vi "main 0.3.vi"() -> ()   [LabVIEW 2012]
uses:
  <vilib>/Utility/file.llb/Write To Spreadsheet File (DBL).vi
  <vilib>/Analysis/1siggen.llb/Ramp Pattern by Samples.vi
  <vilib>/Analysis/NI_AALBase.lvlib
panel:
  in  "stop":bool
  out "Slide":dbl(slide) scale=0.0..1.0
  in  "Tab Control":enum32{"live", "XY"}(tab)
  in  "binning":dbl=4.0
  in  "exp time [s]":dbl=0.01
  in  "frames":i32=1
  in  "avg[t] acc[f]":bool
  in  "threshold":i32=1
  in  "dark?":bool
  in  "dark":bool
  out "Waveform Chart":dbl(graph)=418707489.0
  in  "snap":bool
  in  "count?":bool
  in  "save":bool
  in  "Path":path
  out "XY":dbl[][](graph)
  in  "meas_start_XY":bool
  in  "Axis2":string(combo)="4D Z"
  in  "Axis1":string(combo)="4D Z"
  in  "windows":dbl=1000.0 caption="+/- window" format="%#_6e"
  in  "steps":u32=10
  in  "IP address":string="172.24.192.135"
  in  "meas_stop_XY":bool
  out "captured":dbl[][](graph)
  out "live":dbl[][](graph)
  in  "close":bool
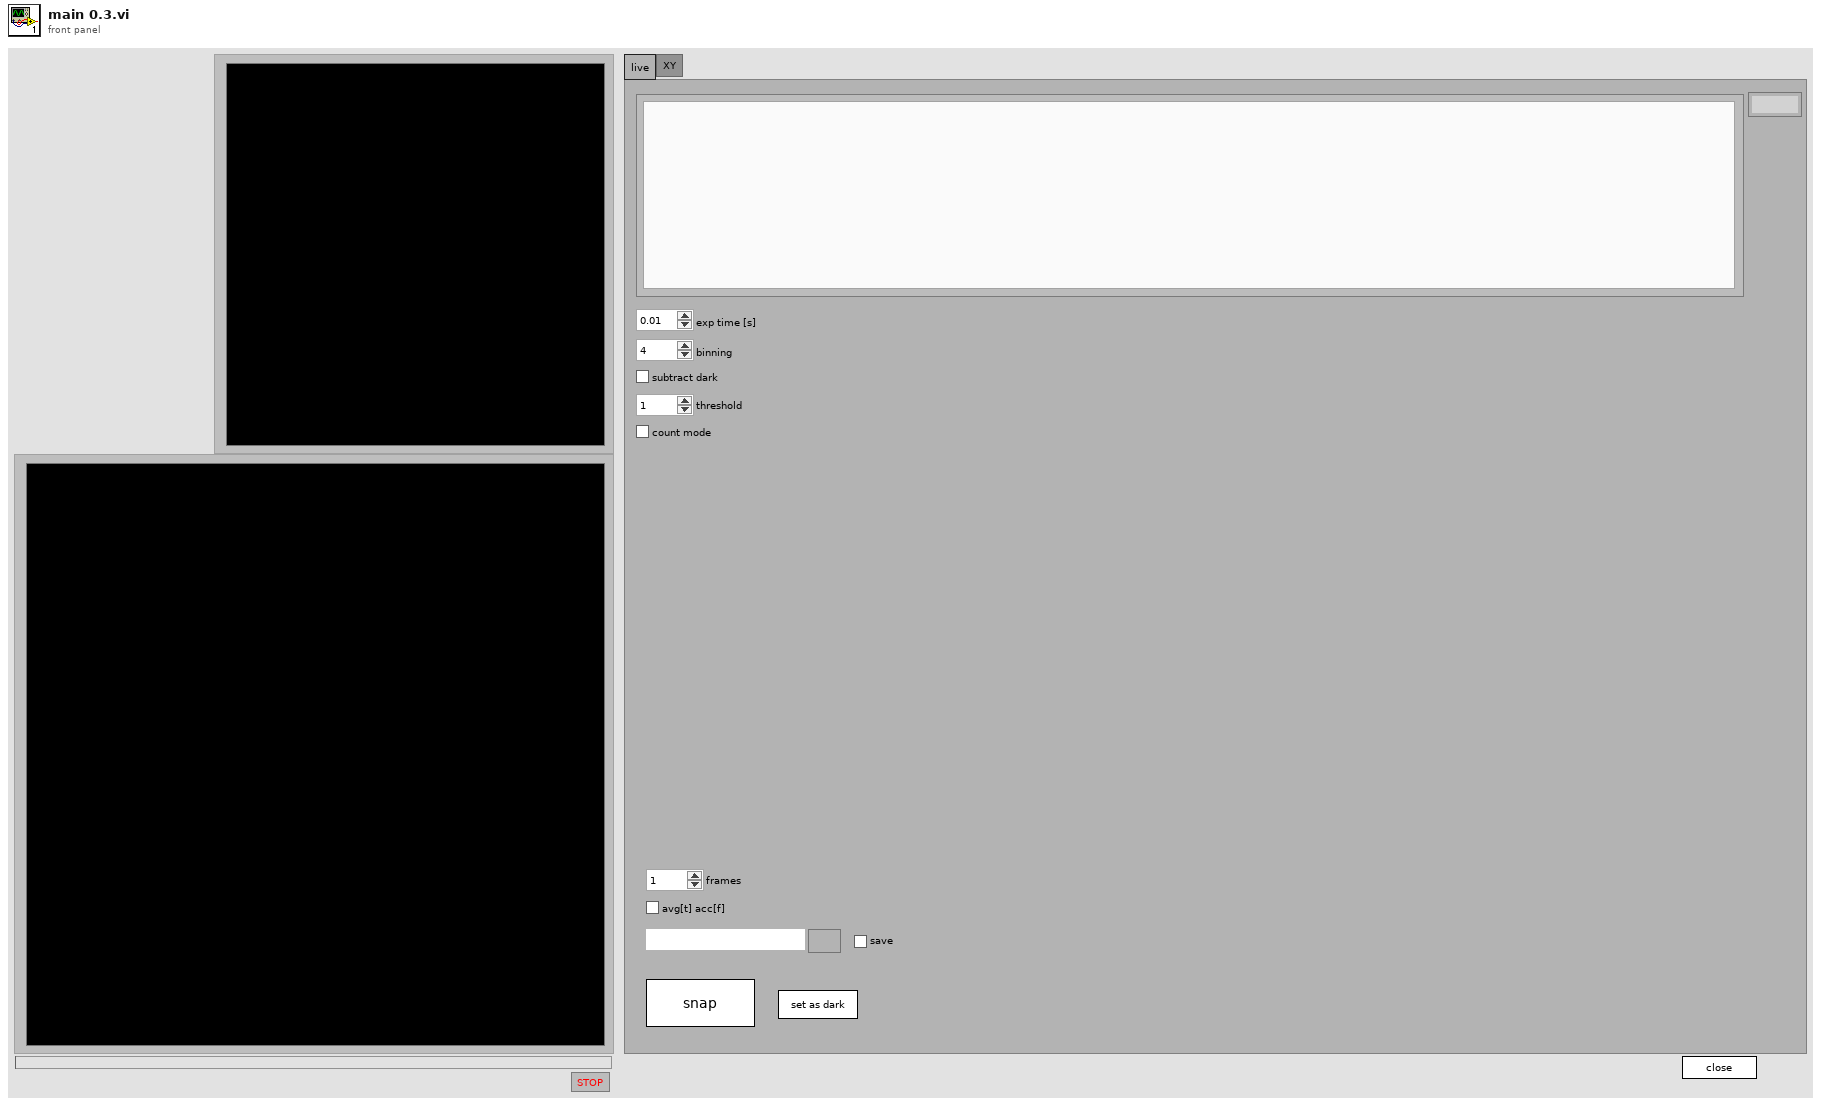
[diagram p1: front panel]
types:
  T1 = cluster{"height":u32, "width":u32, "datatype":u32}
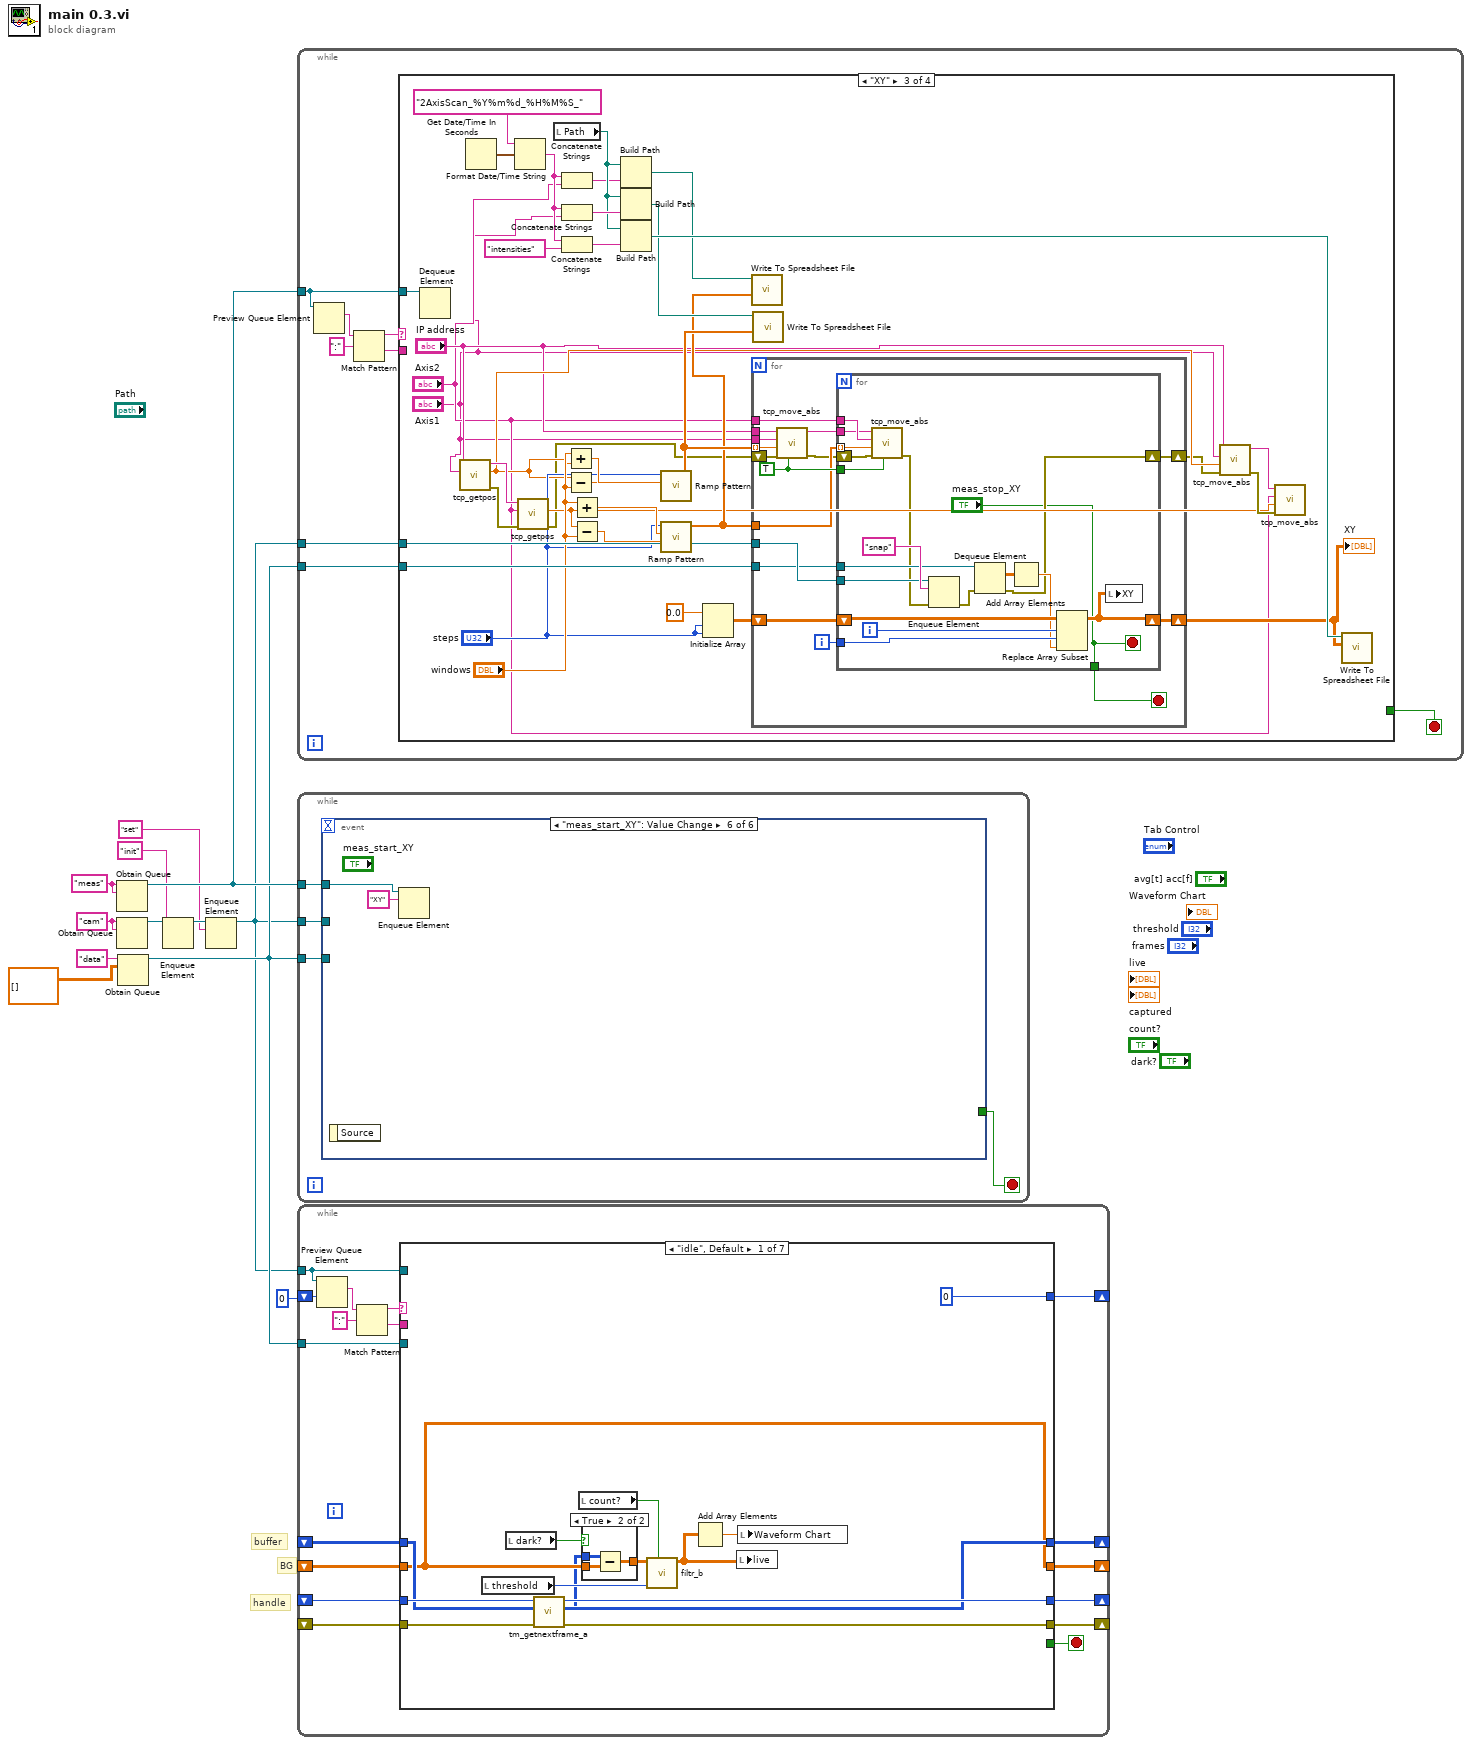
[diagram p0: block diagram]
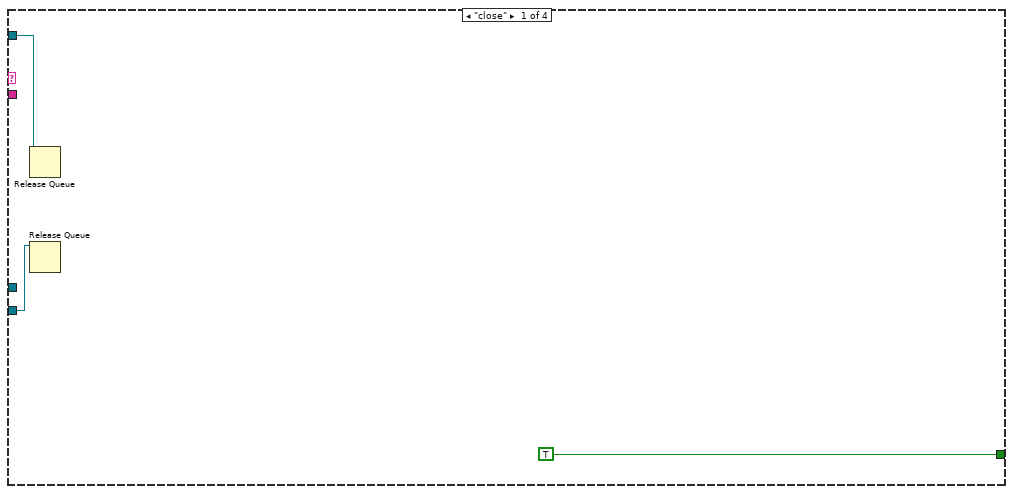
[diagram p2: hidden frame]
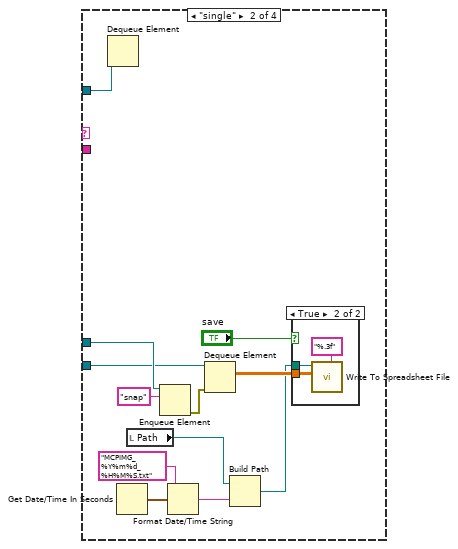
[diagram p3: hidden frame]
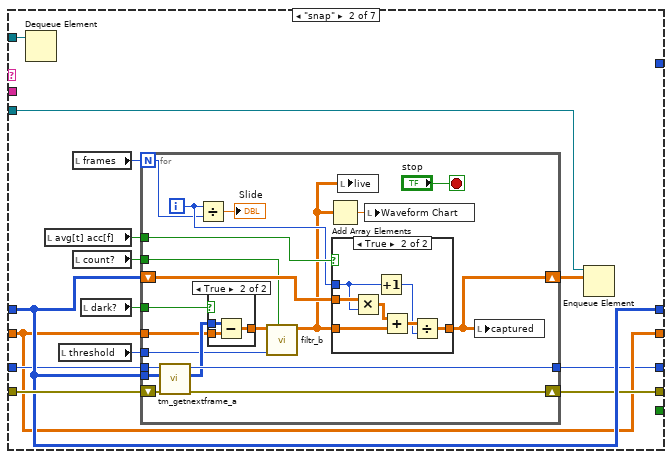
[diagram p7: hidden frame]
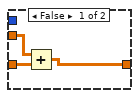
[diagram p8: hidden frame]
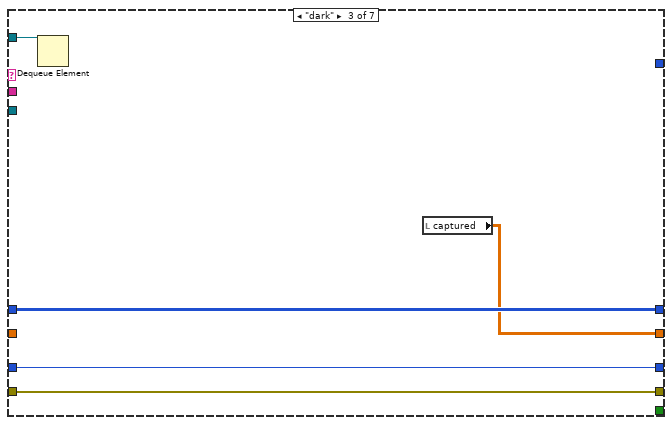
[diagram p10: hidden frame]
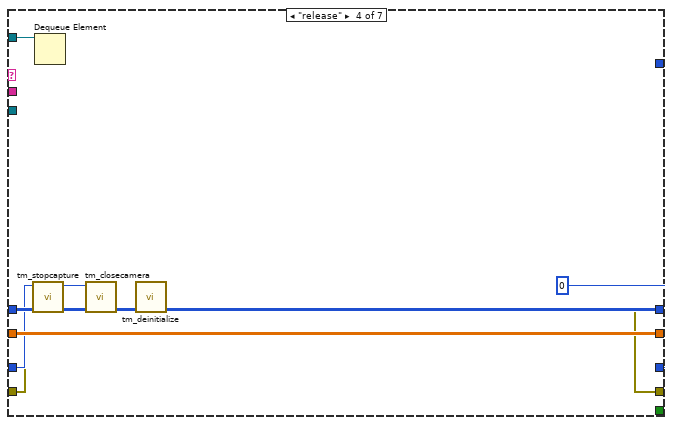
[diagram p11: hidden frame]
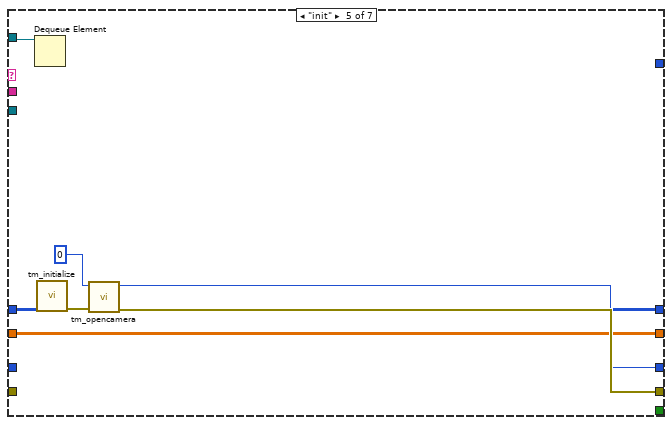
[diagram p12: hidden frame]
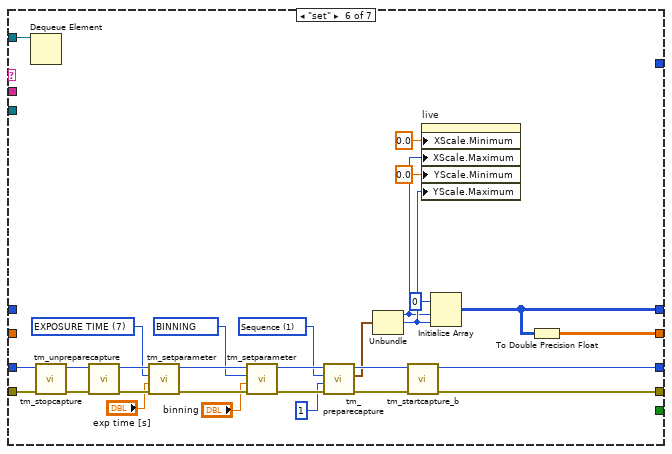
[diagram p13: hidden frame]
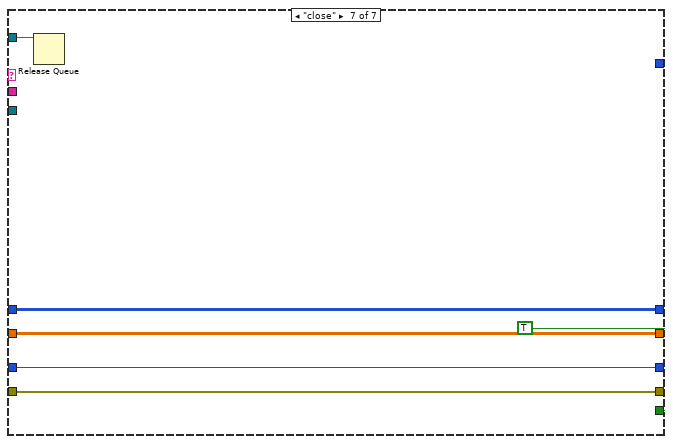
[diagram p14: hidden frame]
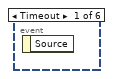
[diagram p15: hidden frame]
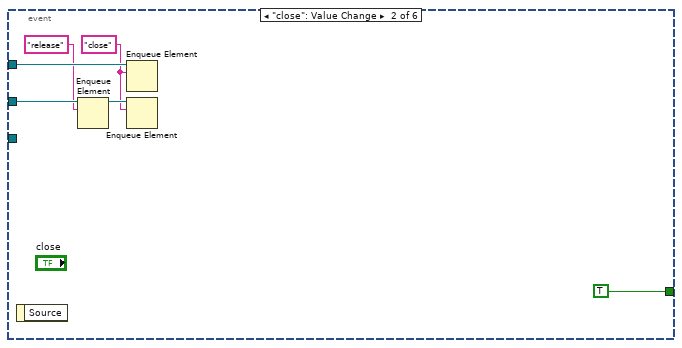
[diagram p16: hidden frame]
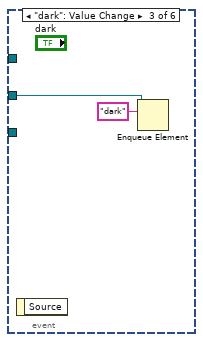
[diagram p17: hidden frame]
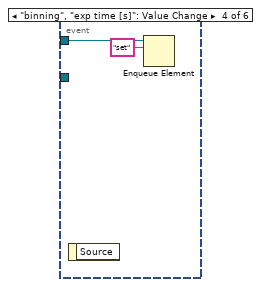
[diagram p18: hidden frame]
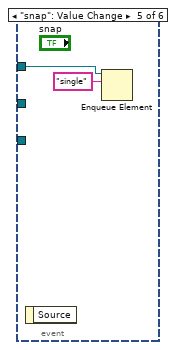
[diagram p19: hidden frame]
diagram:
  w9 = "meas" ("name (unnamed)")
  w10 = "cam" ("name (unnamed)")
  # "BG"
  # "handle"
  # "buffer"
  n1 = Obtain Queue(name (unnamed)=w9, element data type=w9) -> (queue out=w8:refnum<queue>)  [unwired: 3 in, 2 out]
  n2 = Obtain Queue(name (unnamed)=w10, element data type=w10) -> (queue out=w12:refnum<queue>)  [unwired: 3 in, 2 out]
  n3 = Obtain Queue(name (unnamed)="data", element data type=dbl[][] []) -> (queue out=w2:refnum<queue>)  [unwired: 3 in, 2 out]
  n4 = Enqueue Element(queue=w12, element="init") -> (queue out=w6:refnum<queue>)  [unwired: 2 in, 2 out]
  n5 = Enqueue Element(queue=w6, element="set") -> (queue out=w1:refnum<queue>)  [unwired: 2 in, 2 out]
  n6 = while {
    tunnel: w8 -> [w16]
    tunnel: w2 -> [w15]
    tunnel: w1 -> [w13]
    stop <- w14 stop-if-true
    n7 = Preview Queue Element(queue=w16) -> (element=w20:string)  [unwired: 2 in, 3 out]
    n8 = Match Pattern(string=w20, regular expression=":") -> (before substring=w18:string, after substring=w17:string)  [unwired: 1 in, 2 out]
    n9 = case shown="\"XY\"" w18 {
      tunnel: w17 -> [_ _ _ _]
      tunnel: w16 -> [w22 w35 w74 _]
      tunnel: w15 -> [w23 w32 w70 _]
      tunnel: [TRUE _ _ _] -> w14
      tunnel: w13 -> [_ w34 w71 _]
      frame "close" {
        n10 = Release Queue(queue=w22) -> ()  [unwired: 2 in, 3 out]
        n11 = Release Queue(queue=w23) -> ()  [unwired: 2 in, 3 out]
      }
      frame "single" {
        n12 = Dequeue Element(queue=w35) -> ()  [unwired: 2 in, 4 out]
        n13 = Get Date/Time In Seconds() -> (seconds since 1Jan1904=w28:timestamp)
        n14 = local read "Path"() -> (w24:path)
        n15 = Enqueue Element(queue=w34, element="snap") -> (error out=w31:errorcluster)  [unwired: 2 in, 2 out]
        n16 = Format Date/Time String(time format string (%c)="MCPIMG_%Y%m%d_%H%M%S.txt", seconds (now)=w28) -> (date/time string=w26:string)  [unwired: 1 in]
        n17 = Dequeue Element(queue=w32, error in (no error)=w31) -> (element=w30:dbl[][])  [unwired: 1 in, 3 out]
        n18 = Build Path(base path=w24, name or relative path=w26) -> (appended path=w25:path)
        n19 = case shown="True" "save" {
          tunnel: w30 -> [_ w38]
          tunnel: w25 -> [_ w36]
          frame False {
          }
          frame True {
            n20 = call-poly <vilib>:"Write To Spreadsheet File.vi"("format (%.3f)"="%.3f", "2D data"=w38, "file path (dialog if empty)"=w36) -> ()  [unwired: 5 in, 1 out]
          }
        }
      }
      frame "XY" {
        n21 = Dequeue Element(queue=w74) -> ()  [unwired: 2 in, 4 out]
        n22 = call "tcp_getpos.vi"("Axis"="Axis1", "IP address"="IP address") -> ("error out"=w58:errorcluster, "position"=w45:dbl, "IP address out"=w59:string)  [unwired: 7 in]
        n23 = Get Date/Time In Seconds() -> (seconds since 1Jan1904=w69:timestamp)
        n24 = Format Date/Time String(time format string (%c)="2AxisScan_%Y%m%d_%H%M%S_", seconds (now)=w69) -> (date/time string=w53:string)  [unwired: 1 in]
        n25 = call "tcp_getpos.vi"("error in (no error)"=w58, "Axis"="Axis2", "IP address"=w59) -> ("error out"=w39:errorcluster, "position"=w43:dbl)  [unwired: 6 in, 1 out]
        n26 = local read "Path"() -> (w52:path)
        n27 = Concatenate Strings(w53, "Axis2") -> (w51:string)
        n28 = Concatenate Strings(w53, "Axis1") -> (w65:string)
        n29 = Concatenate Strings(w53, "intensities" ("name or relative path")) -> (w66:string)
        n30 = Add(x="windows", y=w45) -> (x+y=w61:dbl)
        n31 = Subtract(x=w45, y="windows") -> (x-y=w60:dbl)
        n32 = Add(x="windows", y=w43) -> (x+y=w56:dbl)
        n33 = Subtract(x=w43, y="windows") -> (x-y=w55:dbl)
        n34 = Build Path(base path=w52, name or relative path=w51) -> (appended path=w50:path)
        n35 = Build Path(base path=w52, name or relative path=w65) -> (appended path=w62:path)
        n36 = Build Path(base path=w52, name or relative path=w66) -> (appended path=w64:path)
        n37 = call-poly <vilib>:"Ramp Pattern.vi"("start"=w60, "end"=w61, "samples"="steps") -> ("Ramp Pattern"=w63:dbl[])  [unwired: 7 in, 1 out]
        n38 = call-poly <vilib>:"Ramp Pattern.vi"("start"=w55, "end"=w56, "samples"="steps") -> ("Ramp Pattern"=w49:dbl[])  [unwired: 7 in, 1 out]
        n39 = Initialize Array(0.0 ("element"), "steps", "steps") -> (w72:dbl[][])
        n40 = call-poly <vilib>:"Write To Spreadsheet File.vi"("1D data"=w49, "file path (dialog if empty)"=w50) -> ()  [unwired: 6 in, 1 out]
        n41 = for {
          tunnel: w63 -> [w90] mode=indexing
          tunnel: "Axis1" -> [w89]
          tunnel: w71 -> [w88]
          tunnel: w70 -> [w87]
          tunnel: "Axis2" -> [w83]
          tunnel: "IP address" -> [w82]
          shift-right: [w81] -> w48
          shift-left: w72 -> [w86]
          tunnel: w49 -> [w80]
          shift-right: [w77] -> w40
          shift-left: w39 -> [w76]
          i -> [w85]
          stop <- w75 stop-if-true
          w84 = TRUE ("wait4motiondone")
          n42 = call "tcp_move_abs.vi"("wait4motiondone"=w84, "error in (no error)"=w76, "destination nm/u°"=w90, "Axis"=w89, "IP address"=w82) -> ("error out"=w79:errorcluster, "IP address out"=w78:string)  [unwired: 4 in, 1 out]
          n43 = for {
            tunnel: w80 -> [w99] mode=indexing
            tunnel: w88 -> [w106]
            tunnel: w87 -> [w105]
            tunnel: w85 -> [w103]
            shift-right: [w93] -> w81
            shift-left: w86 -> [w104]
            tunnel: w84 -> [w97]
            tunnel: w83 -> [w96]
            tunnel: w78 -> [w94]
            shift-right: [w92] -> w77
            shift-left: w79 -> [w95]
            tunnel: ["meas_stop_XY"] -> w75
            i -> [w102]
            stop <- "meas_stop_XY" stop-if-true
            n44 = call "tcp_move_abs.vi"("wait4motiondone"=w97, "error in (no error)"=w95, "destination nm/u°"=w99, "Axis"=w96, "IP address"=w94) -> ("error out"=w98:errorcluster)  [unwired: 4 in, 2 out]
            n45 = Enqueue Element(queue=w106, element="snap", error in (no error)=w98) -> (error out=w107:errorcluster)  [unwired: 1 in, 2 out]
            n46 = Dequeue Element(queue=w105, error in (no error)=w107) -> (element=w101:dbl[][], error out=w92:errorcluster)  [unwired: 1 in, 2 out]
            n47 = Add Array Elements(numeric array=w101) -> (sum=w100:dbl)
            n48 = Replace Array Subset(array=w104, new element=w100, index (row)=w102, index (col)=w103) -> (w93:dbl[][])
            n49 = local write "XY"(w93) -> ()
          }
        }
        "XY" <- w48
        n50 = call-poly <vilib>:"Write To Spreadsheet File.vi"("1D data"=w63, "file path (dialog if empty)"=w62) -> ()  [unwired: 6 in, 1 out]
        n51 = call "tcp_move_abs.vi"("error in (no error)"=w40, "destination nm/u°"=w45, "Axis"="Axis1", "IP address"="IP address") -> ("error out"=w47:errorcluster, "IP address out"=w46:string)  [unwired: 5 in, 1 out]
        n52 = call "tcp_move_abs.vi"("error in (no error)"=w47, "destination nm/u°"=w43, "Axis"="Axis2", "IP address"=w46) -> ()  [unwired: 5 in, 3 out]
        n53 = call-poly <vilib>:"Write To Spreadsheet File.vi"("2D data"=w48, "file path (dialog if empty)"=w64) -> ()  [unwired: 6 in, 1 out]
      }
      frame "idle", Default {
      }
    }
  }
  n54 = while {
    tunnel: w1 -> [w112]
    tunnel: w8 -> [w111]
    tunnel: w2 -> [w110]
    stop <- w109 stop-if-true
    n55 = event shown="[5] \"meas_start_XY\": Value Change" {
      selector: _ -> [_ _ _ _ _ _]
      dyn-events: _ -> [_ _ _ _ _ _]
      timeout: _ -> [_ _ _ _ _ _]
      tunnel: w112 -> [_ w117 w120 w122 _ _]
      tunnel: w111 -> [_ w118 _ _ w123 w125]
      tunnel: w110 -> [_ _ _ _ _ _]
      tunnel: [_ TRUE _ _ _ _] -> w109
      event Timeout {
        n56 = event-data() -> ()  [unwired: 1 in, 1 out]
      }
      event "close": Value Change {
        w114 = "close" ("element")
        n57 = event-data() -> ()  [unwired: 1 in, 1 out]
        n58 = Enqueue Element(queue=w117, element="release") -> (queue out=w116:refnum<queue>)  [unwired: 2 in, 2 out]
        n59 = Enqueue Element(queue=w118, element=w114) -> ()  [unwired: 2 in, 3 out]
        n60 = Enqueue Element(queue=w116, element=w114) -> ()  [unwired: 2 in, 3 out]
      }
      event "dark": Value Change {
        n61 = event-data() -> ()  [unwired: 1 in, 1 out]
        n62 = Enqueue Element(queue=w120, element="dark") -> ()  [unwired: 2 in, 3 out]
      }
      event "binning", "exp time [s]": Value Change {
        n63 = event-data() -> ()  [unwired: 1 in, 1 out]
        n64 = Enqueue Element(queue=w122, element="set") -> ()  [unwired: 2 in, 3 out]
      }
      event "snap": Value Change {
        n65 = event-data() -> ()  [unwired: 1 in, 1 out]
        n66 = Enqueue Element(queue=w123, element="single") -> ()  [unwired: 2 in, 3 out]
      }
      event "meas_start_XY": Value Change {
        n67 = event-data() -> ()  [unwired: 1 in, 1 out]
        n68 = Enqueue Element(queue=w125, element="XY") -> ()  [unwired: 2 in, 3 out]
      }
    }
  }
  n69 = while {
    tunnel: w1 -> [w139]
    shift-right: [w137] -> _
    shift-left: _ -> [w136]
    shift-right: [w135] -> _
    shift-left: _ -> [w134]
    shift-right: [w133] -> _
    shift-left: _ -> [w132]
    shift-right: [w131] -> _
    shift-left: _ -> [w130]
    shift-right: [w128] -> _
    shift-left: 0 -> [w129]
    tunnel: w2 -> [w127]
    stop <- w138 stop-if-true
    n70 = Preview Queue Element(queue=w139, timeout in ms (-1)=w129) -> (element=w143:string)  [unwired: 1 in, 3 out]
    n71 = Match Pattern(string=w143, regular expression=":") -> (before substring=w141:string, after substring=w140:string)  [unwired: 1 in, 2 out]
    n72 = case shown="\"idle\", Default" w141 {
      tunnel: w140 -> [_ _ _ _ _ _ _]
      tunnel: w139 -> [_ w167 w214 w224 w225 w237 w266]
      tunnel: [_ _ _ _ _ _ TRUE] -> w138
      tunnel: [w152 w169 w212 w216 w230 w238 w261] -> w137
      tunnel: w136 -> [w154 w172 w212 w220 _ w260 w261]
      tunnel: [w153 w164 w211 u32 0 ("Handle out") w228 w239 w262] -> w135
      tunnel: w134 -> [w155 w170 w211 w221 _ w258 w262]
      tunnel: [w151 w171 w213 w222 w226 w240 w263] -> w133
      tunnel: w132 -> [w151 w171 w213 w222 w226 _ w263]
      tunnel: [w150 w168 w210 w223 w227 w241 w264] -> w131
      tunnel: w130 -> [w150 w168 _ w223 w227 _ w264]
      tunnel: [0 _ _ _ _ _ _] -> w128
      tunnel: w127 -> [_ w163 _ _ _ _ _]
      frame "idle", Default {
        n73 = local read "threshold"() -> (w156:i32)
        n74 = local read "dark?"() -> (w157:bool)
        n75 = call "tm_getnextframe_a.vi"("error in (no error)"=w154, "Buffer"=w151, "Handle in"=w155) -> ("error out"=w152:errorcluster, "Data"=w148:u16[][], "Handle out"=w153:u32)  [unwired: 6 in]
        n76 = local read "count?"() -> (w146:bool)
        n77 = case shown="True" w157 {
          tunnel: [w158 w161] -> w147
          tunnel: w148 -> [w158 w160]
          tunnel: w150 -> [_ w159]
          frame False {
          }
          frame True {
            n78 = Subtract(x=w160, y=w159) -> (x-y=w161:dbl[][])
          }
        }
        n79 = call "filtr_b.vi"("count?"=w146, "threshold"=w156, "input array"=w147) -> ("output array"=w145:dbl[][])  [unwired: 8 in]
        n80 = Add Array Elements(numeric array=w145) -> (sum=w144:dbl)
        n81 = local write "live"(w145) -> ()
        n82 = local write "Waveform Chart"(w144) -> ()
      }
      frame "snap" {
        n83 = Dequeue Element(queue=w167) -> ()  [unwired: 2 in, 4 out]
        n84 = local read "avg[t] acc[f]"() -> (w166:bool)
        n85 = local read "threshold"() -> (w174:i32)
        n86 = local read "frames"() -> (w173:i32)
        n87 = local read "count?"() -> (w165:bool)
        n88 = local read "dark?"() -> (w175:bool)
        n89 = for {
          N: w173 -> [w180]
          tunnel: w175 -> [w195]
          tunnel: w171 -> [w193]
          tunnel: w170 -> [w194]
          tunnel: w174 -> [w187]
          tunnel: [w191] -> w164
          shift-right: [w190] -> w169
          shift-left: w172 -> [w192]
          tunnel: w168 -> [w186]
          shift-right: [w183] -> w162
          shift-left: w171 -> [w184]
          tunnel: w166 -> [w185]
          tunnel: w165 -> [w182]
          i -> [w181]
          stop <- "stop" stop-if-true
          n90 = call "tm_getnextframe_a.vi"("error in (no error)"=w192, "Buffer"=w193, "Handle in"=w194) -> ("error out"=w190:errorcluster, "Data"=w189:u16[][], "Handle out"=w191:u32)  [unwired: 6 in]
          n91 = Divide(x=w181, y=w180) -> (x/y=→"Slide":dbl)
          n92 = case shown="True" w195 {
            tunnel: [w206 w209] -> w188
            tunnel: w189 -> [w206 w208]
            tunnel: w186 -> [_ w207]
            frame False {
            }
            frame True {
              n93 = Subtract(x=w208, y=w207) -> (x-y=w209:dbl[][])
            }
          }
          n94 = call "filtr_b.vi"("count?"=w182, "threshold"=w187, "input array"=w188) -> ("output array"=w177:dbl[][])  [unwired: 8 in]
          n95 = Add Array Elements(numeric array=w177) -> (sum=w178:dbl)
          n96 = case shown="True" w185 {
            tunnel: w184 -> [w198 w205]
            tunnel: w177 -> [w197 w203]
            tunnel: [w196 w199] -> w183
            tunnel: w181 -> [_ w200]
            frame False {
              n97 = Add(x=w198, y=w197) -> (x+y=w196:dbl[][])
            }
            frame True {
              n98 = Multiply(x=w205, y=w200) -> (x*y=w204:dbl[][])
              n99 = Increment(x=w200) -> (x+1=w201:i32)
              n100 = Add(x=w204, y=w203) -> (x+y=w202:dbl[][])
              n101 = Divide(x=w202, y=w201) -> (x/y=w199:dbl[][])
            }
          }
          n102 = local write "live"(w177) -> ()
          n103 = local write "Waveform Chart"(w178) -> ()
          n104 = local write "captured"(w183) -> ()
        }
        n105 = Enqueue Element(queue=w163, element=w162) -> ()  [unwired: 2 in, 3 out]
      }
      frame "dark" {
        n106 = Dequeue Element(queue=w214) -> ()  [unwired: 2 in, 4 out]
        n107 = local read "captured"() -> (w210:dbl[][])
      }
      frame "release" {
        n108 = call "tm_stopcapture.vi"("error in (no error)"=w220, "Handle in"=w221) -> ("error out"=w218:errorcluster, "Handle out"=w219:u32)  [unwired: 8 in]
        n109 = Dequeue Element(queue=w224) -> ()  [unwired: 2 in, 4 out]
        n110 = call "tm_closecamera.vi"("error in (no error)"=w218, "Handle in"=w219) -> ("error out"=w217:errorcluster)  [unwired: 9 in]
        n111 = call "tm_deinitialize.vi"("error in (no error)"=w217) -> ("error out"=w216:errorcluster)  [unwired: 10 in]
      }
      frame "init" {
        n112 = Dequeue Element(queue=w225) -> ()  [unwired: 2 in, 4 out]
        n113 = call "tm_initialize.vi"() -> ("error out"=w231:errorcluster)  [unwired: 8 in, 3 out]
        n114 = call "tm_opencamera.vi"("error in (no error)"=w231, "Camera Index"=u32 0) -> ("error out"=w230:errorcluster, "Handle out"=w228:u32)  [unwired: 7 in, 1 out]
      }
      frame "set" {
        w246 = 1 items=["Snap", "Sequence"] ("Capture mode")
        w250 = u32 4215968 items=["BINNING"=4215968, "BITS PER CHANNEL"=2, "ACTIVE VIEW INDEX"=3, "CCD MODE"=4, "SENSOR MODE"=5, "READOUT MODE"=6, "EXPOSURE TIME"=7, "CONTRAST GAIN"=8, "CONTRAST OFFSET"=9, "LIGHT MODE"=10, "SENSITIVITY"=11, "WHITE BALANCE"=12, "PHOTON IMAGING MODE"=13, "HIGH DYNAMIC RANGE MODE"=14, "TRIGGER SOURCE"=15, "TRIGGER ACTIVE"=16, "TRIGGER MODE"=17, "TRIGGER POLARITY"=18, "TRIGGER GLOBAL EXPOSURE"=19, "FIRST TRIGGER BEHAVIOR"=20, "TRIGGER TIMES"=21, "OUTPUT TRIGGER POLARITY"=22, "OUTPUT TRIGGER DELAY"=23, "OUTPUT TRIGGER PERIOD"=24, "TEMPERATURE"=25, "TEMPERATURE TARGET"=26, "SENSOR COOLER FAN"=27, "MECHANICAL SHUTTER"=28, "BACK FOCUS POSITION"=29, "FRAMEBUNDLE MODE"=30, "FRAMEBUNDLE NUMBER"=31, "LINEBUNDLE HEIGHT"=32, "TRIGGER CONNECTOR"=33, "IMAGE PIXEL TYPE"=34, "OUTPUT TRIGGER KIND"=35, "READOUT DIRECTION"=36, "CHANNEL SYNC"=37] ("Parameter")
        w254 = u32 7 items=["BINNING"=4215968, "BITS PER CHANNEL"=2, "ACTIVE VIEW INDEX"=3, "CCD MODE"=4, "SENSOR MODE"=5, "READOUT MODE"=6, "EXPOSURE TIME"=7, "CONTRAST GAIN"=8, "CONTRAST OFFSET"=9, "LIGHT MODE"=10, "SENSITIVITY"=11, "WHITE BALANCE"=12, "PHOTON IMAGING MODE"=13, "HIGH DYNAMIC RANGE MODE"=14, "TRIGGER SOURCE"=15, "TRIGGER ACTIVE"=16, "TRIGGER MODE"=17, "TRIGGER POLARITY"=18, "TRIGGER GLOBAL EXPOSURE"=19, "FIRST TRIGGER BEHAVIOR"=20, "TRIGGER TIMES"=21, "OUTPUT TRIGGER POLARITY"=22, "OUTPUT TRIGGER DELAY"=23, "OUTPUT TRIGGER PERIOD"=24, "TEMPERATURE"=25, "TEMPERATURE TARGET"=26, "SENSOR COOLER FAN"=27, "MECHANICAL SHUTTER"=28, "BACK FOCUS POSITION"=29, "FRAMEBUNDLE MODE"=30, "FRAMEBUNDLE NUMBER"=31, "LINEBUNDLE HEIGHT"=32, "TRIGGER CONNECTOR"=33, "IMAGE PIXEL TYPE"=34, "OUTPUT TRIGGER KIND"=35, "READOUT DIRECTION"=36, "CHANNEL SYNC"=37] ("Parameter")
        n115 = Dequeue Element(queue=w237) -> ()  [unwired: 2 in, 4 out]
        n116 = call "tm_stopcapture.vi"("error in (no error)"=w260, "Handle in"=w258) -> ("error out"=w259:errorcluster, "Handle out"=w257:u32)  [unwired: 8 in]
        n117 = call "tm_unpreparecapture.vi"("error in (no error)"=w259, "Handle in"=w257) -> ("error out"=w256:errorcluster, "Handle out"=w255:u32)  [unwired: 8 in]
        n118 = call "tm_setparameter.vi"("error in (no error)"=w256, "Value in"="exp time [s]", "Parameter"=w254, "Handle in"=w255) -> ("error out"=w251:errorcluster, "Handle out"=w252:u32)  [unwired: 6 in]
        n119 = call "tm_setparameter.vi"("error in (no error)"=w251, "Value in"="binning", "Parameter"=w250, "Handle in"=w252) -> ("error out"=w247:errorcluster, "Handle out"=w248:u32)  [unwired: 6 in]
        n120 = call "tm_preparecapture.vi"("error in (no error)"=w247, "Frames"=1, "Capture mode"=w246, "Handle in"=w248) -> ("error out"=w243:errorcluster, "Buffer Info"=w242:T1, "Handle out"=w244:u32)  [unwired: 4 in, 1 out]
        n121 = Unbundle(w242) -> ("height"=w235:u32, "width"=w236:u32)  [unwired: 1 out]
        n122 = call "tm_startcapture_b.vi"("error in (no error)"=w243, "Handle in"=w244) -> ("error out"=w238:errorcluster, "Handle out"=w239:u32)  [unwired: 8 in]
        n123 = property on="live" class="IntGraph (strict)"("XScale.Minimum"=0.0 ("X Scale.Range:Minimum"), "XScale.Maximum"=w235, "YScale.Minimum"=0.0 ("Y Scale.Range:Minimum"), "YScale.Maximum"=w236) -> ()  [unwired: 2 in, 2 out]
        n124 = Initialize Array(u16 0 ("element"), w235, w236) -> (w240:u16[][])
        n125 = To Double Precision Float(number=w240) -> (double precision float=w241:dbl[][])
      }
      frame "close" {
        n126 = Release Queue(queue=w266) -> ()  [unwired: 2 in, 3 out]
      }
    }
  }
